vi "XOR Encryption - (3) Using Separate Keys to Send a Shared Key.vi"() -> ()   [LabVIEW 2013]
panel:
  out "Data Out":string
  in  "Data In":string
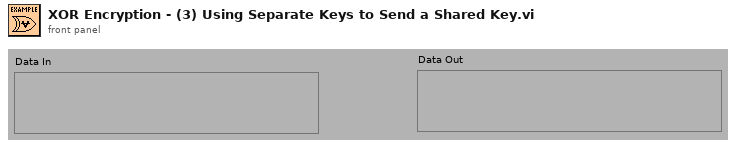
[diagram p1: front panel]
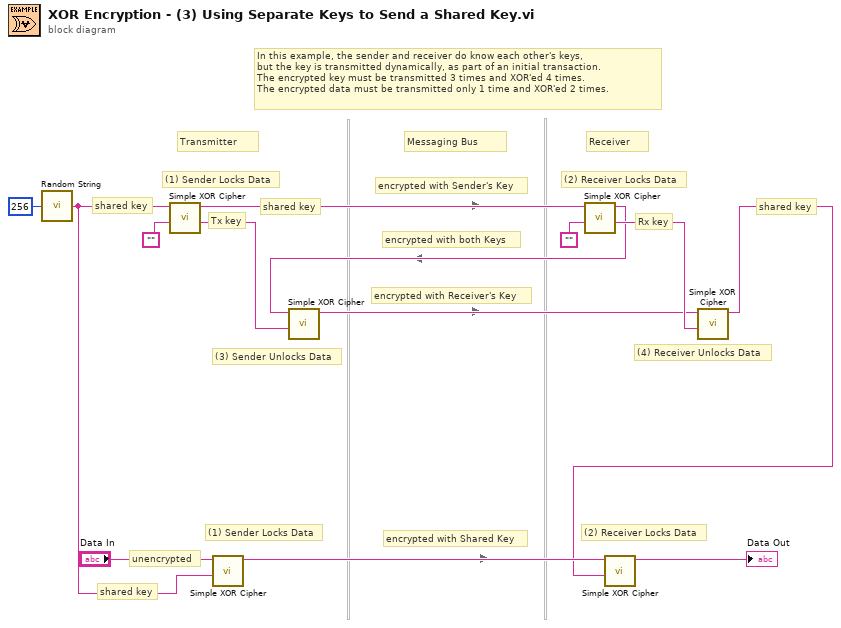
[diagram p0: block diagram]
diagram:
  # "shared key"
  # "shared key"
  # "shared key"
  # "unencrypted"
  # "encrypted with Shared Key"
  # "(2) Receiver Locks Data"
  # "(1) Sender Locks Data"
  # "Messaging Bus"
  # "Receiver"
  # "Transmitter"
  # "shared key"
  # "Rx key"
  # "Tx key"
  # "In this example, the sender and receiver do know each other's keys,\nbut the key is transmitted dynamically, as part of an initial transaction.\nThe encrypted key must be transmitted 3 times and XOR'ed 4 times.\nThe encrypted data must be transmitted only 1 time and XOR'ed 2 times."
  # "encrypted with Receiver's Key"
  # "encrypted with Sender's Key"
  # "encrypted with both Keys"
  # "(4) Receiver Unlocks Data"
  # "(3) Sender Unlocks Data"
  # "(2) Receiver Locks Data"
  # "(1) Sender Locks Data"
  n1 = call "Random String.vi"("length"=256) -> ("random data"=w2:string)  [unwired: 4 in]
  n2 = call "Simple XOR Cipher.vi"("key (\"\": random)"="", "data in"=w2) -> ("key out"=w12:string, "data out"=w10:string)  [unwired: 8 in]
  n3 = call "Simple XOR Cipher.vi"("key (\"\": random)"=w2, "data in"="Data In") -> ("data out"=w6:string)  [unwired: 8 in, 1 out]
  n4 = call "Simple XOR Cipher.vi"("key (\"\": random)"="", "data in"=w10) -> ("key out"=w13:string, "data out"=w8:string)  [unwired: 8 in]
  n5 = call "Simple XOR Cipher.vi"("key (\"\": random)"=w12, "data in"=w8) -> ("data out"=w9:string)  [unwired: 8 in, 1 out]
  n6 = call "Simple XOR Cipher.vi"("key (\"\": random)"=w13, "data in"=w9) -> ("data out"=w1:string)  [unwired: 8 in, 1 out]
  n7 = call "Simple XOR Cipher.vi"("key (\"\": random)"=w1, "data in"=w6) -> ("data out"=→"Data Out":string)  [unwired: 8 in, 1 out]
